vi "pid array element to object test.vi"() -> ()   [LabVIEW 2014, in "Tagbus PID Module tests.lvlib"]
uses:
  Tagbus PID Module tests.lvlib
  editor node/PID array element.ctl
  module/configuration/PID Loop.lvclass
  module/configuration/PID Loop/PID Parameters.ctl
  module/configuration/PID Loop/PID Gains.ctl
  module/configuration/PID Loop/PID Range.ctl
  editor node/Tagbus PID Module editor node.lvclass
panel:
  out "output range":T1={"output high"=100.0, "output low"=-100.0} {"output low" format="%.2f"; "output high" format="%.2f"}
  out "PID gains":T2={"proportional gain (Kc)"=1.0, "integral time (Ti, min)"=0.01, "derivative time (Td, min)"=0.0} {"proportional gain (Kc)" format="%.2f"; "integral time (Ti, min)" format="%.2f"}
  out "PID Parameters":T3
  out "ID":string
  out "error out":errorcluster
  out "reference out":refnum<class "PID Loop.lvclass">
  in  "error in (no error)":errorcluster
  in  "PID Element in":T4
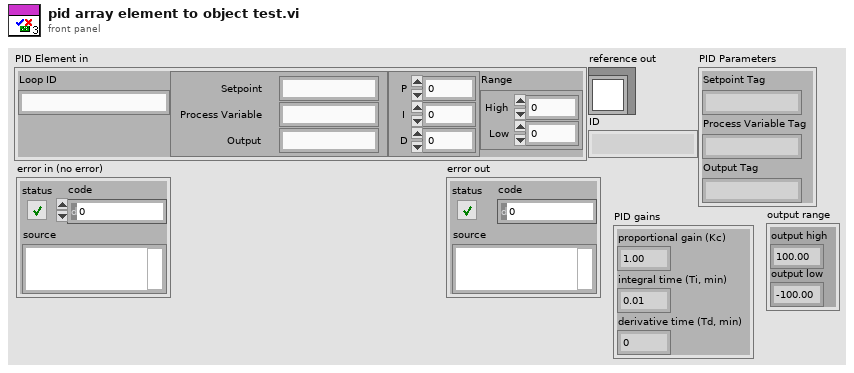
[diagram p1: front panel]
types:
  T1 = typedef "PID Loop.lvclass/PID Range.ctl" = cluster{"output high":dbl, "output low":dbl}
  T2 = typedef "PID Loop.lvclass/PID Gains.ctl" = cluster{"proportional gain (Kc)":dbl, "integral time (Ti, min)":dbl, "derivative time (Td, min)":dbl}
  T3 = typedef "PID Loop.lvclass/PID Parameters.ctl" = cluster{"Setpoint Tag":string, "Process Variable Tag":string, "Output Tag":string}
  T4 = typedef "Tagbus PID Module editor node.lvclass/PID array element.ctl" = cluster{"Loop ID":string, "Tags":cluster{"Setpoint":string, "Process Variable":string, "Output":string}, "Gains":cluster{"P":dbl, "I":dbl, "D":dbl}, "Range":cluster{"High":dbl, "Low":dbl}}
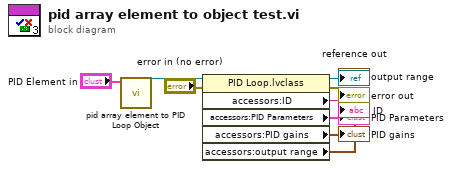
[diagram p0: block diagram]
diagram:
  n1 = call "pid array element to PID Loop Object.vi"("PID Element in"="PID Element in") -> ("PID Loop out"=w8:refnum<class "PID Loop.lvclass">)  [unwired: 9 in, 1 out]
  n2 = property class="PID Loop.lvclass"(reference=w8, error in="error in (no error)") -> (reference out=→"reference out":refnum<class "PID Loop.lvclass">, error out=→"error out":errorcluster, "accessors:ID"=→"ID":string, "accessors:PID Parameters"=→"PID Parameters":T3, "accessors:PID gains"=→"PID gains":T2, "accessors:output range"=→"output range":T1)
